vi "GetSceneBoundaries.vi"(8 "error in":errorcluster, 11 "class data in":refnum<class "SceneRoot.lvclass">) -> (0 "error out":errorcluster, 2 "boundaries out":T1, 3 "class data out":refnum<class "SceneRoot.lvclass">)   [LabVIEW 2010, in "RenderBase.lvlib" / "SceneRoot.lvclass"]
doc: "Returns the scene boundaries."
uses:
  SceneRoot.lvclass
  <vilib>/Utility/miscctls.llb/LVPoint32TypeDef.ctl
  SceneRoot.lvclass/SceneRoot.ctl
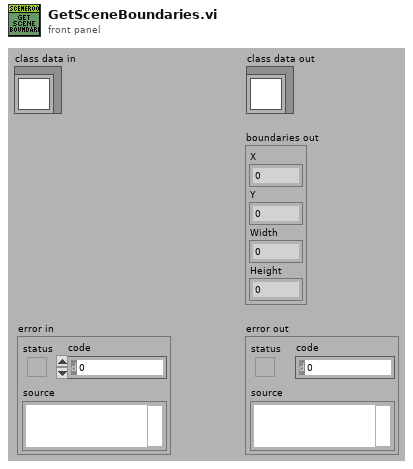
[diagram p1: front panel]
types:
  T1 = cluster{"X":sgl, "Y":sgl, "Width":sgl, "Height":sgl}
  T2 = typedef "LVPoint32TypeDef.ctl" = cluster{"Horizontal":i32, "Vertical":i32}
  T3 = typedef "LVBoundsTypeDef.ctl" = cluster{"Width":u32, "Height":u32}
  T4 = typedef "LV3DPointTypeDef.ctl" = cluster{"X":sgl, "Y":sgl, "Z":sgl}
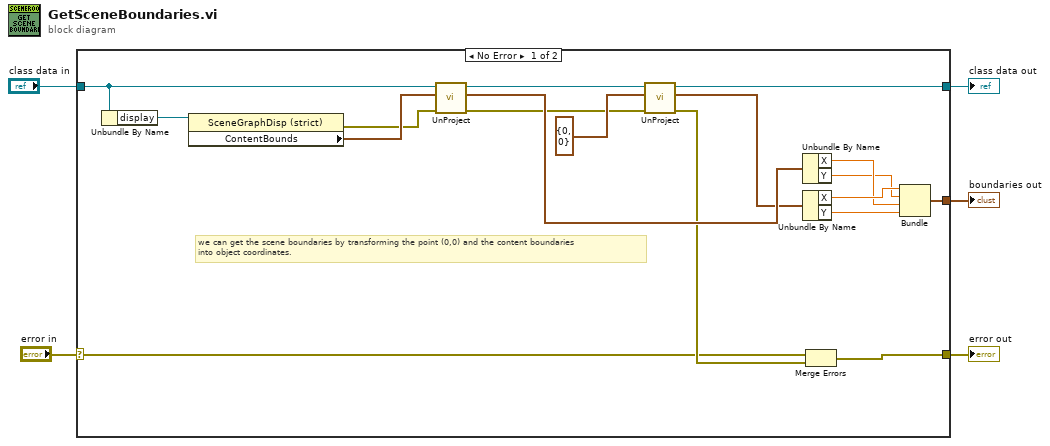
[diagram p0: block diagram]
diagram:
  n1 = case shown="No Error" "error in" {
    selector: "error in" -> [w6 w25]
    tunnel: [w23 _] -> w5
    tunnel: [w7 w25] -> w3
    tunnel: [w12 w24] -> w1
    tunnel: "class data in" -> [w17 w24]
    frame No Error {
      # "we can get the scene boundaries by transforming the point (0,0) and the content boundaries\ninto object coordinates."
      n2 = Unbundle By Name(w17) -> ("display"=w18:refnum<vi>)
      n3 = property on="Property Node" class="SceneGraphDisp (strict)"(reference=w18) -> (error out=w14:errorcluster, "ContentBounds"=w15:T3)  [unwired: 1 in, 1 out]
      n4 = call "UnProject.vi"("error in"=w14, "winCoords in"=w15, "class data in"=w17) -> ("error out"=w10:errorcluster, "sceneCoords out"=w13:T4, "class data out"=w16:refnum<class "SceneRoot.lvclass">)  [unwired: 6 in]
      n5 = call "UnProject.vi"("error in"=w10, "winCoords in"=T2 {"Horizontal"=0, "Vertical"=0} ("point"), "class data in"=w16) -> ("error out"=w8:errorcluster, "sceneCoords out"=w9:T4, "class data out"=w12:refnum<class "SceneRoot.lvclass">)  [unwired: 6 in]
      n6 = Unbundle By Name(w13) -> ("X"=w21:sgl, "Y"=w20:sgl)
      n7 = Unbundle By Name(w9) -> ("X"=w22:sgl, "Y"=w19:sgl)
      n8 = Merge Errors(w6, w8) -> (w7:errorcluster)
      n9 = Bundle("X"=w22, "Y"=w20, "X"=w21, "Y"=w19) -> (w23:cluster{"X":sgl, "Y":sgl, "X":sgl, "Y":sgl})  [unwired: 1 in]
    }
    frame Error {
    }
  }
  "boundaries out" <- w5
  "error out" <- w3
  "class data out" <- w1
